vi "wymus blad.vi"(11 "error in (no error)":errorcluster) -> (3 "error out":errorcluster)   [LabVIEW 2014]
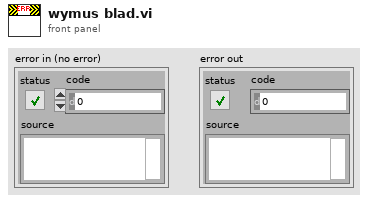
[diagram p1: front panel]
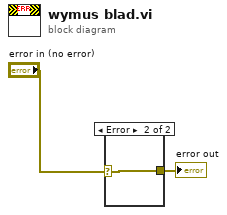
[diagram p0: block diagram]
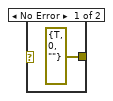
[diagram p2: hidden frame]
diagram:
  n1 = case shown="Error" "error in (no error)" {
    selector: "error in (no error)" -> [_ w4]
    tunnel: [errorcluster {"status"=TRUE, "code"=0, "source"=""} ("error in") w4] -> w2
    frame No Error {
    }
    frame Error {
    }
  }
  "error out" <- w2
